vi "lfieldpanel_DO_stream_frames.vi"(5 "savepath":path, 7 "Log data":bool, 8 "error in (no error)":errorcluster, 9 "stop_stream":refnum<notifier>, 10 "Integrate_sensor":bool, 11 "lightfield_panel in":refnum<class "lightfield_panel.lvclass">) -> (0 "error out":errorcluster, 3 "lightfield_panel out":refnum<class "lightfield_panel.lvclass">)   [LabVIEW 2015, in "lightfield_panel.lvclass"]
uses:
  lightfield_panel.lvclass
  lightfield/lightfield_class.lvclass
  UI/panel_class/panel.lvclass
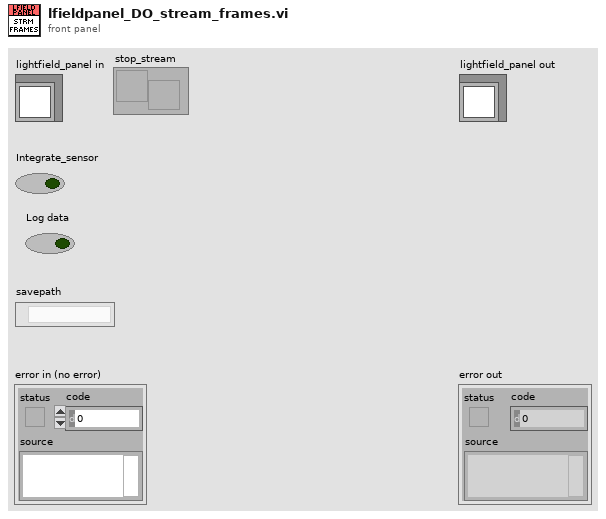
[diagram p1: front panel]
types:
  T1 = cluster{"Image":dbl[][][], "Frame Size":cluster{"F":i32, "Y":i32, "X":i32}}
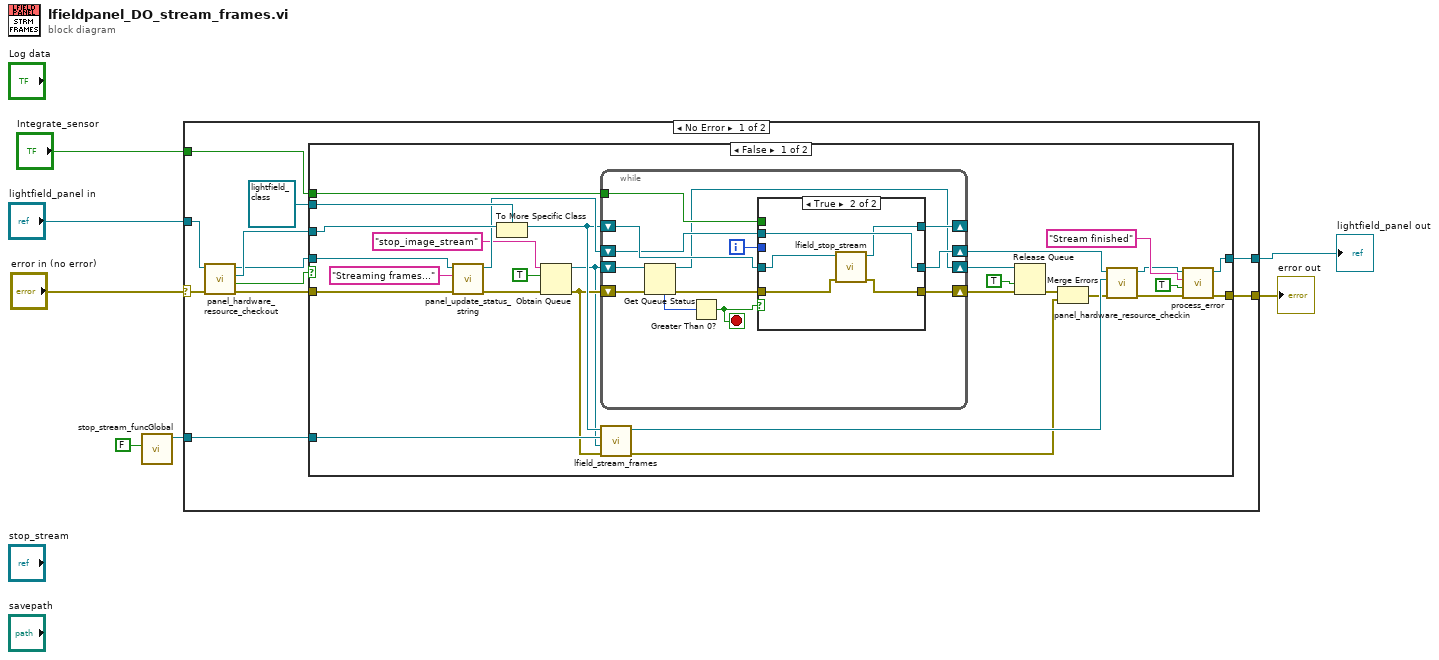
[diagram p0: block diagram]
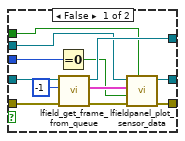
[diagram p2: hidden frame]
diagram:
  n1 = call "stop_stream_funcGlobal.vi"("write?"=FALSE) -> ("queue out 2"=w1:refnum<queue>)  [unwired: 10 in]
  n2 = case shown="No Error" "error in (no error)" {
    selector: "error in (no error)" -> [w18 w80]
    tunnel: [w12 w80] -> w4
    tunnel: [w11 w79] -> w6
    tunnel: "lightfield_panel in" -> [w10 w79]
    tunnel: "Integrate_sensor" -> [w9 _]
    tunnel: w1 -> [w8 _]
    frame No Error {
      n3 = call "panel_hardware_resource_checkout.vi"("error in (no error)"=w18, "panel in"=w10) -> ("error out"=w14:errorcluster, "timed out?"=w17:bool, "hardware.lvclass"=w15:refnum<class "hardware.lvclass">, "panel out"=w13:refnum<class "lightfield_panel.lvclass">)  [unwired: 6 in]
      n4 = case shown="False" w17 {
        tunnel: refnum<class "lightfield_class.lvclass"> refnum ("lightfield_class.lvclass") -> [w46 _]
        tunnel: w15 -> [w45 _]
        tunnel: w14 -> [w39 w77]
        tunnel: w13 -> [w38 w78]
        tunnel: [w43 w77] -> w12
        tunnel: [w42 w78] -> w11
        tunnel: w9 -> [w30 _]
        tunnel: w8 -> [w28 _]
        frame False {
          n5 = call-dynamic "panel_update_status_string.vi"("error in (no error)"=w39, "String"="Streaming frames...", "lightfield_panel in"=w38) -> ("error out"=w27:errorcluster, "lightfield_panel out"=w35:refnum<class "lightfield_panel.lvclass">)  [unwired: 7 in]
          n6 = To More Specific Class(target class=w46, reference=w45) -> (specific class reference=w34:refnum<class "lightfield_class.lvclass">)  [unwired: 1 in, 1 out]
          n7 = Obtain Queue(name (unnamed)="stop_image_stream", element data type=TRUE, error in (no error)=w27) -> (queue out=w23:refnum<queue>, error out=w26:errorcluster)  [unwired: 2 in, 1 out]
          n8 = while {
            shift-right: [w55] -> w22
            shift-left: w26 -> [w52]
            shift-right: [w49] -> w20
            shift-left: w23 -> [w50]
            shift-right: [w57] -> w31
            shift-left: w35 -> [w56]
            shift-right: [w58] -> _
            shift-left: w34 -> [w59]
            tunnel: w30 -> [w53]
            i -> [w54]
            stop <- w47 stop-if-true
            n9 = Get Queue Status(queue=w50, error in (no error)=w52) -> (queue out=w49:refnum<queue>, error out=w51:errorcluster, # elements in queue=w48:i32)  [unwired: 1 in, 5 out]
            n10 = Greater Than 0?(x=w48) -> (x > 0?=w47:bool)
            n11 = case shown="True" w47 {
              tunnel: w59 -> [w70 w73]
              tunnel: [w69 w72] -> w58
              tunnel: [w68 w76] -> w57
              tunnel: w56 -> [w67 w76]
              tunnel: [w66 w74] -> w55
              tunnel: w54 -> [w64 _]
              tunnel: w53 -> [w62 _]
              tunnel: w51 -> [w61 w75]
              frame False {
                n12 = Equal To 0?(x=w64) -> (x = 0?=w63:bool)
                n13 = call "lfield_get_frame_from_queue.vi"("error in (no error)"=w61, "timeout"=-1, "lightfield_class in"=w70) -> ("error out"=w71:errorcluster, "image_data"=w65:T1, "lightfield_class out"=w69:refnum<class "lightfield_class.lvclass">)  [unwired: 6 in]
                n14 = call "lfieldpanel_plot_sensor_data.vi"("Integrate"=w62, "error in (no error)"=w71, "First_time?"=w63, "image_data"=w65, "lightfield_panel in"=w67) -> ("error out"=w66:errorcluster, "lightfield_panel out"=w68:refnum<class "lightfield_panel.lvclass">)  [unwired: 5 in]
              }
              frame True {
                n15 = call "lfield_stop_stream.vi"("error in (no error)"=w75, "lightfield_class in"=w73) -> ("error out"=w74:errorcluster, "lightfield_class out"=w72:refnum<class "lightfield_class.lvclass">)  [unwired: 8 in]
              }
            }
          }
          n16 = call "lfield_stream_frames.vi"("error in (no error)"=w26, "stop_image_stream"=w23, "stop_stream_queue"=w28, "lightfield_class in"=w34) -> ("error out"=w33:errorcluster, "lightfield_class out"=w36:refnum<class "lightfield_class.lvclass">)  [unwired: 6 in]
          n17 = Release Queue(queue=w20, force destroy? (F)=TRUE, error in (no error)=w22) -> (error out=w21:errorcluster)  [unwired: 2 out]
          n18 = Merge Errors(w21, w33) -> (w32:errorcluster)
          n19 = call "panel_hardware_resource_checkin.vi"("error in (no error)"=w32, "hardware.lvclass"=w36, "panel in"=w31) -> ("error out"=w44:errorcluster, "panel out"=w29:refnum<class "lightfield_panel.lvclass">)  [unwired: 7 in]
          n20 = call "process_error.vi"("error in (no error)"=w44, "Update Status"=TRUE, "No Error Message"="Stream finished", "lightfield_panel in"=w29) -> ("error out"=w43:errorcluster, "lightfield_panel out"=w42:refnum<class "lightfield_panel.lvclass">)  [unwired: 6 in]
        }
        frame True {
        }
      }
    }
    frame Error {
    }
  }
  "error out" <- w4
  "lightfield_panel out" <- w6
